vi "Test Messdaten erzeugen.vi"(7 "Anzahl Werte":i32=5) -> (2 "Messdaten":sgl[](array[numeric]))   [LabVIEW 2020, in "CAN Interface.lvlib"]
uses:
  CAN Interface.lvlib
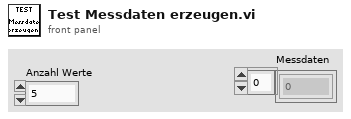
[diagram p1: front panel]
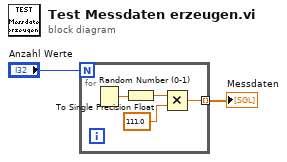
[diagram p0: block diagram]
diagram:
  n1 = for {
    N: "Anzahl Werte" -> [_]
    tunnel: [w3] -> w1 mode=indexing
    n2 = Random Number (0-1)() -> (number: 0 to 1=w5:dbl)
    n3 = To Single Precision Float(number=w5) -> (single precision float=w4:sgl)
    n4 = Multiply(x=w4, y=sgl 111.0) -> (x*y=w3:sgl)
  }
  "Messdaten" <- w1
